vi "test-ElevatorSim.vi"() -> (3 "Test Passed":bool)   [LabVIEW 2019]
uses:
  <vilib>/Rock Robotics/WPI/ThirdParty/JAS_Junk/TrajLib/DCMOTOR.CTL
  <vilib>/Rock Robotics/WPI/ThirdParty/JAS_Junk/TrajLib/ELEVATOR_SIM.ctl
  <vilib>/Rock Robotics/WPI/ThirdParty/JAS_Junk/TrajLib/LINEAR_SYSTEM_SIM.ctl
  <vilib>/Rock Robotics/WPI/ThirdParty/JAS_Junk/TrajLib/LINEAR_SYSTEM.ctl
  <vilib>/Analysis/Matrix/Datatypes/RealMatrix.ctl
  <vilib>/Rock Robotics/WPI/ThirdParty/JAS_Junk/TrajLib/PID_ERROR_TOLERANCE.ctl
  <vilib>/Rock Robotics/WPI/ThirdParty/JAS_Junk/TrajLib/DCMotor_New.vi
  <vilib>/Rock Robotics/WPI/ThirdParty/JAS_Junk/TrajLib/Units_RotationsPerMinuteToRadiansPerSecond.vi
  <vilib>/Rock Robotics/WPI/ThirdParty/JAS_Junk/TrajLib/MatBuilder_Create.vi
  <vilib>/Rock Robotics/WPI/ThirdParty/JAS_Junk/TrajLib/PIDController_Calculate_SP_PV.vi
  <vilib>/Rock Robotics/WPI/ThirdParty/JAS_Junk/TrajLib/PIDController_AtSetpoint.vi
  <vilib>/Rock Robotics/WPI/ThirdParty/JAS_Junk/TrajLib/PIDController_SetPID.vi
  <vilib>/Rock Robotics/WPI/ThirdParty/JAS_Junk/TrajLib/PIDController_SetIntegratorRange.vi
  <vilib>/Rock Robotics/WPI/ThirdParty/JAS_Junk/TrajLib/PIDController_SetTolerancePandV.vi
  <vilib>/Rock Robotics/WPI/ThirdParty/JAS_Junk/TrajLib/PIDController_DisableContinousInput.vi
  <vilib>/Rock Robotics/WPI/ThirdParty/JAS_Junk/TrajLib/PIDController_EnableContinousInput.vi
  <vilib>/Rock Robotics/WPI/ThirdParty/JAS_Junk/TrajLib/PIDController_Reset.vi
  <vilib>/Rock Robotics/WPI/ThirdParty/JAS_Junk/TrajLib/PIDController_NewPeriod.vi
  <vilib>/Rock Robotics/WPI/ThirdParty/JAS_Junk/TrajLib/BatterySim_CalculateLoadedBatteryVoltage.vi
  <vilib>/Rock Robotics/WPI/ThirdParty/JAS_Junk/TrajLib/PIDController_SetSetpoint.vi
  <vilib>/Rock Robotics/WPI/ThirdParty/JAS_Junk/TrajLib/PIDController_Calculate_PV.vi
  <vilib>/Rock Robotics/WPI/ThirdParty/JAS_Junk/TrajLib/ControllerUtil_GetModulusError.vi
  <vilib>/Rock Robotics/SystemInterfaces/NetworkCommunication/NetComm_UsageReport_report.vi
  <vilib>/Rock Robotics/WPI/ThirdParty/JAS_Junk/TrajLib/Util_LibraryGlobals.vi
  <vilib>/Rock Robotics/WPI/ThirdParty/JAS_Junk/TrajLib/Trajectory_Library.lvlib
  <vilib>/Analysis/Matrix/NI_Matrix.lvlib
panel:
  in  "Tab Control":enum32{"Page 2", "Page 6", "Page 7"}(tab)
  out "Elevator Motor":T1 {"Jr_KgM2" format="%13.5p"; "L_H" format="%13.5p"; "Kt_NMPerAmp" format="%13.5p"; "KvINV_RadPerSecPerVolt" format="%13.5p"; "R_Ohms" format="%13.5p"; "FreeSpeed_RadPerSec" format="%13.5p"; "FreeCurrent_Amps" format="%13.5p"; "StallCurrent_Amps" format="%13.5p"; "StallTorque_NM" format="%13.5p"; "nominalVoltage_Volts" format="%13.5p"}
  out "Elevator Simulaation":T2 {"GearBox"."Jr_KgM2" format="%13.5p"; "GearBox"."L_H" format="%13.5p"; "GearBox"."Kt_NMPerAmp" format="%13.5p"; "GearBox"."KvINV_RadPerSecPerVolt" format="%13.5p"; "GearBox"."R_Ohms" format="%13.5p"; "GearBox"."FreeSpeed_RadPerSec" format="%13.5p"; "GearBox"."FreeCurrent_Amps" format="%13.5p"; "GearBox"."StallCurrent_Amps" format="%13.5p"; "GearBox"."StallTorque_NM" format="%13.5p"; "GearBox"."nominalVoltage_Volts" format="%13.5p"}
  out "Motor Out":cluster{"Voltage":dbl}(graph)
  out "PV Chart":cluster{dbl}(graph)
  out "At Top":bool
  out "At Bottom":bool
  in  "SP-SetPoint":dbl=2.0
  out "AtSetpoint":bool
  out "CO-ControlOutput":dbl
  out "Voltage":dbl
  out "Position_Meters":dbl
  # "<States, 1>"
  # "<Outputs, 1>"
  # "<Inputs, 1>"
  # "<Outputs, 1>"
  # "<States,States>"
  # "<States,Inputs>"
  # "<Outputs,States>"
  # "<Outputs,Inputs>"
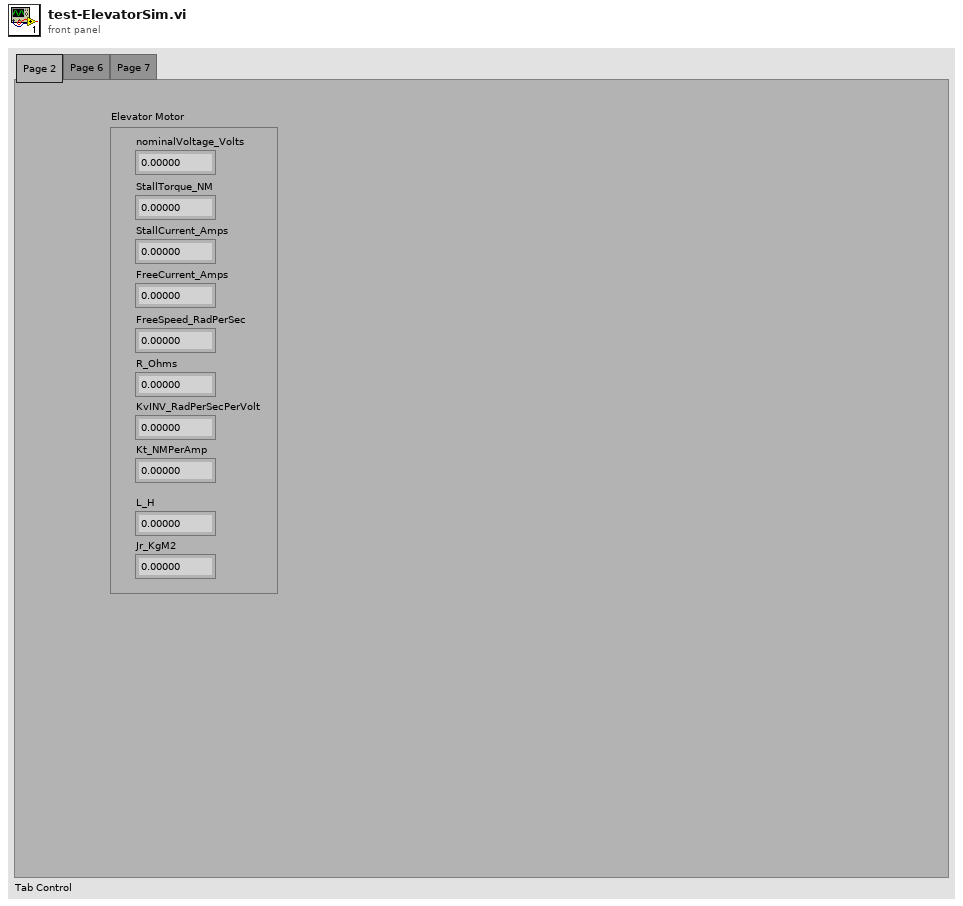
[diagram p1: front panel]
types:
  T1 = typedef "Trajectory_Library.lvlib/DCMOTOR.CTL" = cluster{"nominalVoltage_Volts":dbl, "StallTorque_NM":dbl, "StallCurrent_Amps":dbl, "FreeCurrent_Amps":dbl, "FreeSpeed_RadPerSec":dbl, "R_Ohms":dbl, "KvINV_RadPerSecPerVolt":dbl, "Kt_NMPerAmp":dbl, "L_H":dbl, "Jr_KgM2":dbl}
  T2 = typedef "Trajectory_Library.lvlib/ELEVATOR_SIM.ctl" = cluster{"LinearSystemSim":T3, "GearBox":T1, "Gearing":dbl, "DrumRadius_M":dbl, "MinHeight_M":dbl, "MaxHeight_M":dbl, "CarriageMass_Kg":dbl}
  T3 = typedef "Trajectory_Library.lvlib/LINEAR_SYSTEM_SIM.ctl" = cluster{"m_Plant":T4, "m_X":T5, "m_Y":T5, "m_U":T5, "MeasureStdDev":T5}
  T4 = typedef "Trajectory_Library.lvlib/LINEAR_SYSTEM.ctl" = cluster{"m_A":T5, "m_B":T5, "m_C":T5, "m_D":T5, "States":i32, "Inputs":i32, "Outputs":i32}
  T5 = typedef "NI_Matrix.lvlib/RealMatrix.ctl" = dbl[][]
  T6 = typedef "Trajectory_Library.lvlib/PID_ERROR_TOLERANCE.ctl" = cluster{"PositionTolerance":dbl, "VelocityTolerance":dbl}
  T7 = typedef "Trajectory_Library.lvlib/PID_TUNING.ctl" = cluster{"Kp":dbl, "Ki":dbl, "Kd":dbl, "MaximumIntegral":dbl, "MinimumIntegral":dbl}
  T8 = typedef "Trajectory_Library.lvlib/PID_INPUT_LIMITS.ctl" = cluster{"MaxInput":dbl, "MinInput":dbl, "Continuous":bool}
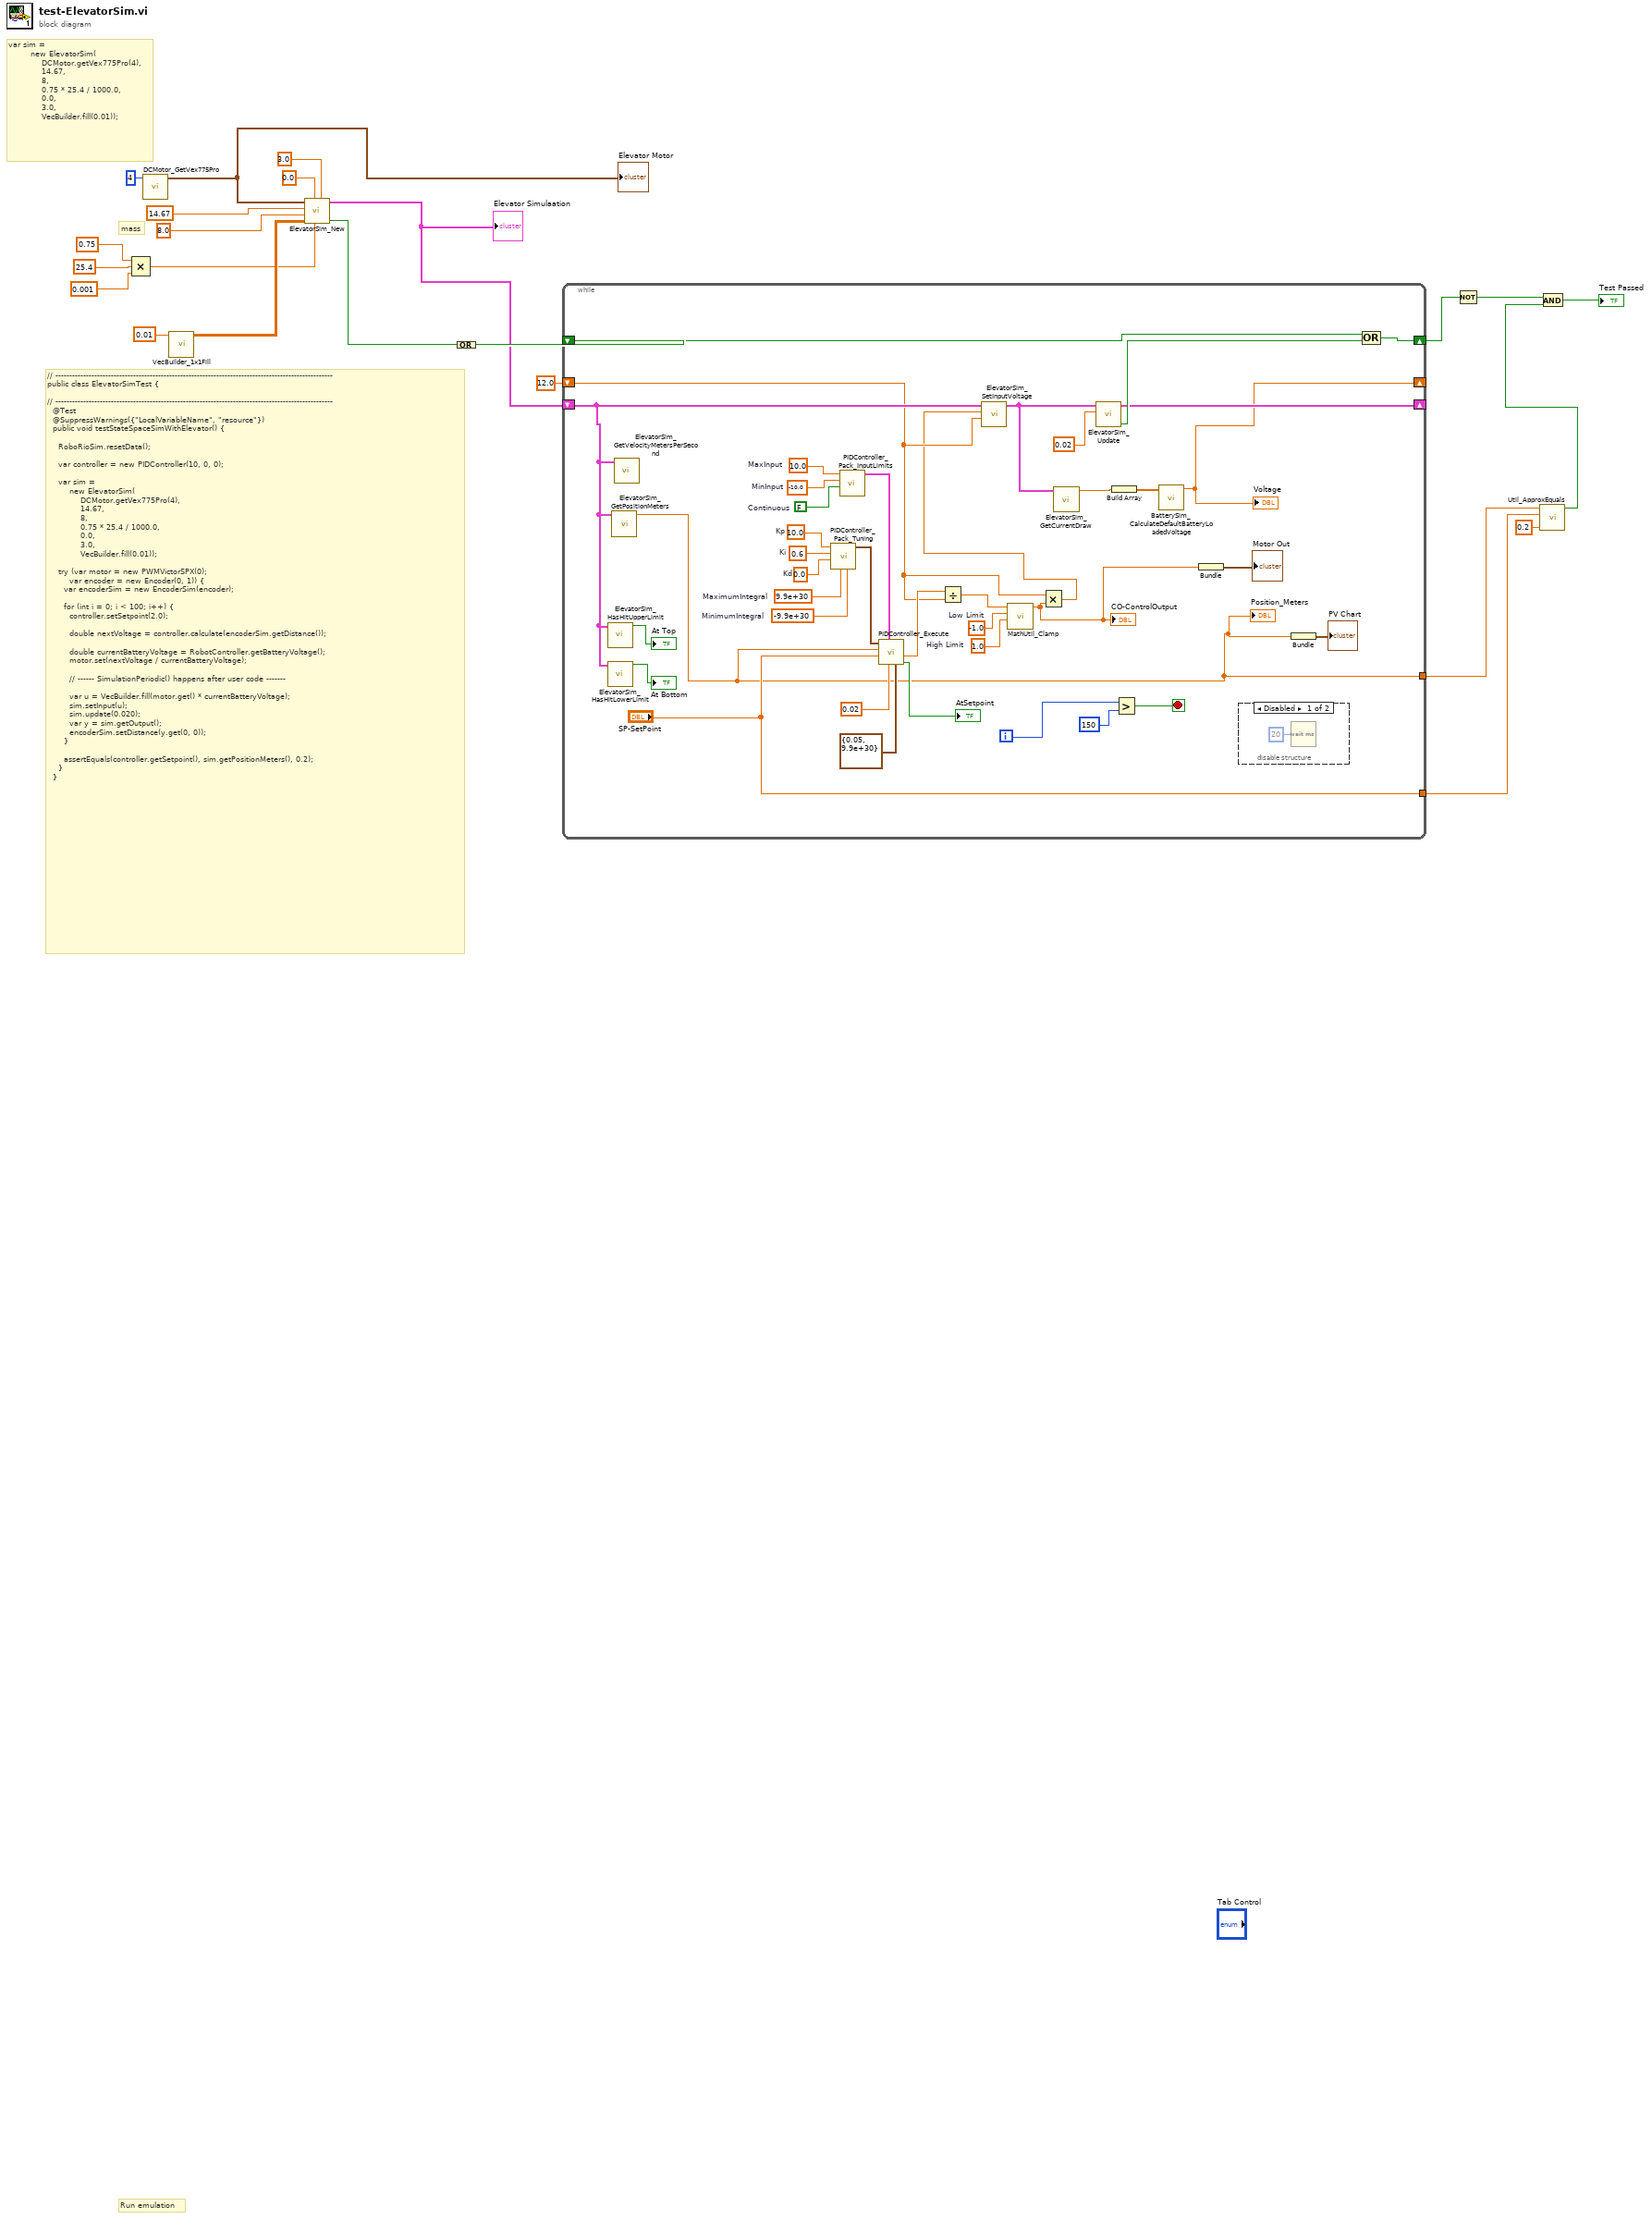
[diagram p0: block diagram]
diagram:
  # "var sim =\n        new ElevatorSim(\n            DCMotor.getVex775Pro(4),\n            14.67,\n            8,\n            0.75 * 25.4 / 1000.0,\n            0.0,\n            3.0,\n            VecBuilder.fill(0.01));"
  # "mass"
  # "// ----------------------------------------------------------------------------------------------------\npublic class ElevatorSimTest {\n\n// ----------------------------------------------------------------------------------------------------\n  @Test\n  @SuppressWarnings({\"LocalVariableName\", \"resource\"})\n  public void testStateSpaceSimWithElevator() {\n\n    RoboRioSim.resetData();\n\n    var controller = new PIDController(10, 0, 0);\n\n    var sim =\n        new ElevatorSim(\n            DCMotor.getVex775Pro(4),\n            14.67,\n            8,\n            0.75 * 25.4 / 1000.0,\n            0.0,\n            3.0,\n            VecBuilder.fill(0.01));\n\n    try (var motor = new PWMVictorSPX(0);\n        var encoder = new Encoder(0, 1)) {\n      var encoderSim = new EncoderSim(encoder);\n\n      for (int i = 0; i < 100; i++) {\n        controller.setSetpoint(2.0);\n\n        double nextVoltage = controller.calculate(encoderSim.getDistance());\n\n        double currentBatteryVoltage = RobotController.getBatteryVoltage();\n        motor.set(nextVoltage / currentBatteryVoltage);\n\n        // ------ SimulationPeriodic() happens after user code -------\n\n        var u = VecBuilder.fill(motor.get() * currentBatteryVoltage);\n        sim.setInput(u);\n        sim.update(0.020);\n        var y = sim.getOutput();\n        encoderSim.setDistance(y.get(0, 0));\n      }\n\n      assertEquals(controller.getSetpoint(), sim.getPositionMeters(), 0.2);\n    }\n  }"
  # "Run emulation"
  n1 = Compound Arithmetic op=MULTIPLY(0.75 ("value"), 25.4 ("value"), 0.001 ("value")) -> (w11:dbl)
  n2 = call <vilib>:"DCMotor_GetVex775Pro.vi"("Num Motors"=4) -> ("DCMOTOR"=w15:T1)  [unwired: 10 in]
  "Elevator Motor" <- w15
  n3 = call <vilib>:"VecBuilder_1x1Fill.vi"("R0_C0"=0.01) -> ("output matrix"=w12:T5)  [unwired: 10 in]
  n4 = call <vilib>:"ElevatorSim_New.vi"("MaxHeight_Meters"=3.0, "DrumRadius_Meters"=w11, "MinHeight_Meters"=0.0, "MeasurementStdDev"=w12, "CarriageMass_Kg"=8.0 ("G"), "Gearing"=14.67, "GearBox"=w15) -> ("Error"=w10:bool, "ElevatorSim"=w9:T2)  [unwired: 3 in]
  "Elevator Simulaation" <- w9
  n5 = Compound Arithmetic op=OR(w10) -> (w21:bool)
  n6 = while {
    shift-right: [w53] -> _
    shift-left: w9 -> [w41]
    shift-right: [w54] -> w2
    shift-left: w21 -> [w55]
    shift-right: [w35] -> _
    shift-left: 12.0 ("Voltage") -> [w30]
    tunnel: ["SP-SetPoint"] -> w5
    tunnel: [w27] -> w6
    i -> [w59]
    stop <- w57 stop-if-true
    w34 = 1.0  # High Limit
    w33 = -1.0  # Low Limit
    w51 = 10.0  # MaxInput
    w50 = -10.0  # MinInput
    w49 = FALSE  # Continuous
    w48 = 10.0  # Kp
    w47 = 0.6  # Ki
    w46 = 0.0  # Kd
    w45 = 9.9e+30  # MaximumIntegral
    w44 = -9.9e+30  # MinimumIntegral
    n7 = call <vilib>:"ElevatorSim_HasHitUpperLimit.vi"("ElevatorSim"=w41) -> ("At HIgh LImit"=→"At Top":bool)  [unwired: 10 in]
    n8 = call <vilib>:"ElevatorSim_HasHitLowerLimit.vi"("ElevatorSim"=w41) -> ("AtLowLimit"=→"At Bottom":bool)  [unwired: 10 in]
    n9 = call <vilib>:"ElevatorSim_GetPositionMeters.vi"("ElevatorSim"=w41) -> ("Position_Meters"=w27:dbl)  [unwired: 10 in]
    "Position_Meters" <- w27
    n10 = call <vilib>:"ElevatorSim_GetVelocityMetersPerSecond.vi"("ElevatorSim"=w41) -> ()  [unwired: 10 in, 1 out]
    n11 = call <vilib>:"PIDController_Pack_Tuning.vi"("MinimumIntegral"=w44, "MaximumIntegral"=w45, "Kd"=w46, "Ki"=w47, "Kp"=w48) -> ("PID Tuning"=w43:T7)  [unwired: 6 in]
    n12 = call <vilib>:"PIDController_Pack_InputLimits.vi"("Continuous"=w49, "MinInput"=w50, "MaxInput"=w51) -> ("PID Input Limits"=w42:T8)  [unwired: 8 in]
    n13 = call <vilib>:"PIDController_Execute.vi"("PID Error Tolerance"=T6 {"PositionTolerance"=0.05, "VelocityTolerance"=9.9e+30}, "Period"=0.02, "PID Input Limits"=w42, "SP-SetPoint"="SP-SetPoint", "PV-Measurement"=w27, "PID Tuning"=w43) -> ("AtSetpoint"=→"AtSetpoint":bool, "CO-ControlOutput"=w32:dbl)  [unwired: 3 in, 1 out]
    n14 = Divide(x=w32, y=w30) -> (x/y=w31:dbl)
    n15 = call <vilib>:"MathUtil_Clamp.vi"("High Limit"=w34, "Low Limit"=w33, "Value"=w31) -> ("Result"=w24:dbl)  [unwired: 8 in]
    "CO-ControlOutput" <- w24
    n16 = Multiply(x=w30, y=w24) -> (x*y=w26:dbl)
    n17 = call <vilib>:"ElevatorSim_SetInputVoltage.vi"("Battery_Volts"=w30, "Input_Voltage"=w26, "in ElevatorSim"=w41) -> ("out ElevatorSim"=w38:T2)  [unwired: 8 in]
    n18 = call <vilib>:"ElevatorSim_GetCurrentDraw.vi"("ElevatorSim"=w38) -> ("Current_Amps"=w37:dbl)  [unwired: 10 in]
    n19 = call <vilib>:"ElevatorSim_Update.vi"("dT_Seconds"=0.02, "in ElevatorSim"=w38) -> ("Error"=w56:bool, "out ElevatorSim"=w53:T2)  [unwired: 8 in]
    n20 = Build Array(w37) -> (w36:dbl[])
    n21 = Greater?(x=w59, y=150) -> (0:w57:bool)
    n22 = call <vilib>:"BatterySim_CalculateDefaultBatteryLoadedVoltage.vi"("Currents"=w36) -> ("Voltage"=w35:dbl)  [unwired: 10 in]
    "Voltage" <- w35
    n23 = Bundle("Result"=w24) -> (→"Motor Out":cluster{"Result":dbl})  [unwired: 1 in]
    n24 = disable-structure shown="Disabled" {
      frame Disabled {
        n25 = Wait (ms)(milliseconds to wait=u32 20) -> ()  [unwired: 1 out]
      }
      frame Enabled {
      }
    }
    n26 = Bundle("Position_Meters"=w27) -> (→"PV Chart":cluster{"Position_Meters":dbl})  [unwired: 1 in]
    n27 = Compound Arithmetic op=OR(w55, w56) -> (w54:bool)
  }
  n28 = Not(x=w2) -> (.not. x?=w1:bool)
  n29 = call <vilib>:"Util_ApproxEquals.vi"("Tolerance"=0.2, "Value 2"=w5, "Value 1"=w6) -> ("ApproxEquals"=w3:bool)  [unwired: 8 in]
  n30 = Compound Arithmetic op=AND(w1, w3) -> (→"Test Passed":bool)
